vi "fs (rate).vi"(0 "Waveform":waveform(dbl), 11 "error in (no error)":errorcluster) -> (4 "period":dbl format="%.2g", 6 "f":dbl, 8 "rpm":dbl, 10 "fs (rate)":dbl, 15 "error out":errorcluster)   [LabVIEW 2013]
uses:
  <vilib>/measure/mascope.llb/Pulse Measurements 1 chan.vi
  <vilib>/measure/NI_MAPro.lvlib
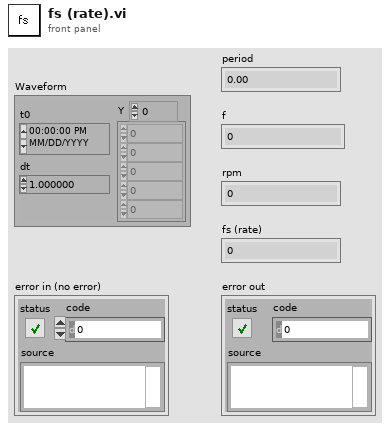
[diagram p1: front panel]
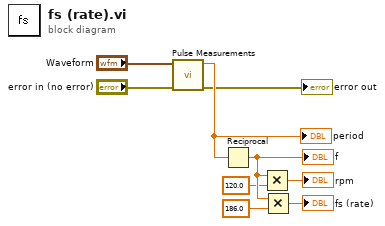
[diagram p0: block diagram]
diagram:
  n1 = call-poly <vilib>:"Pulse Measurements.vi"("error in (no error)"="error in (no error)", "signal in"="Waveform") -> ("error out"=→"error out":errorcluster, "period"=w5:dbl)  [unwired: 5 in, 3 out]
  "period" <- w5
  n2 = Reciprocal(x=w5) -> (1/x=w6:dbl)
  "f" <- w6
  n3 = Multiply(x=w6, y=120.0) -> (x*y=→"rpm":dbl)
  n4 = Multiply(x=w6, y=186.0) -> (x*y=→"fs (rate)":dbl)
